vi "Write Remote UI.vi"(10 "Remote UI":refnum<class "Message Enqueuer.lvclass">, 11 "Controller in":refnum<class "Controller.lvclass">) -> (3 "Controller out":refnum<class "Controller.lvclass">)   [LabVIEW 2011, in "Controller.lvclass"]
uses:
  Controller.lvclass
  <userlib>/_Frameworks/ActorFramework/Message Enqueuer/Message Enqueuer.lvclass
  Controller.lvclass/Controller.ctl
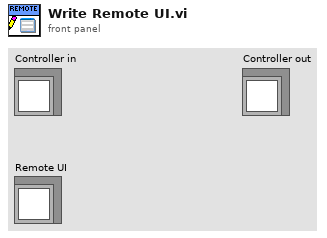
[diagram p1: front panel]
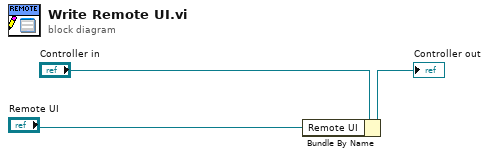
[diagram p0: block diagram]
diagram:
  n1 = Bundle By Name(cluster="Controller in", "Remote UI"="Remote UI") -> (→"Controller out":refnum<class "Controller.lvclass">)
